vi "Test 1.vi"(8 "error in (no error)":errorcluster, 11 "Test Case In":refnum<class "Tests.lvclass">) -> (0 "error out":errorcluster, 3 "Test Case Out":refnum<class "Tests.lvclass">)   [LabVIEW 2021, in "Tests.lvclass"]
uses:
  Tests.lvclass
  C:/Program Files (x86)/National Instruments/LabVIEW 2021/vi.lib/Astemes/LUnit/Test Case.lvclass
  <vilib>/Astemes/LUnit/Test Case.lvclass/Test Case.ctl
  <vilib>/Astemes/LUnit/Append Fail Result.vi
  <vilib>/Astemes/LUnit/Append Pass Result.vi
  Proto/Hailstone.lvclass
  <vilib>/Astemes/LUnit/Test Case.lvclass
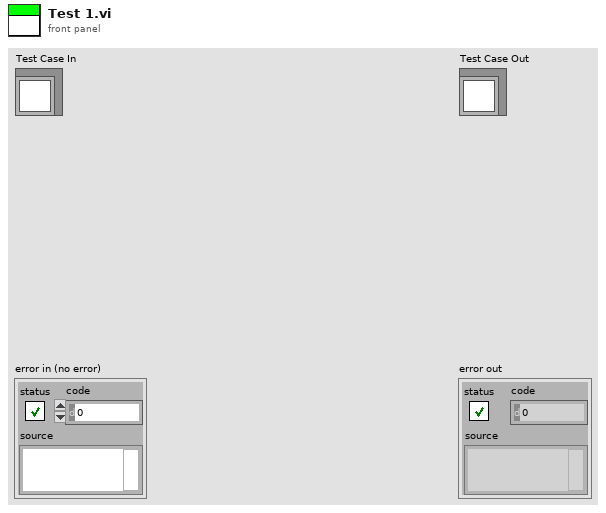
[diagram p1: front panel]
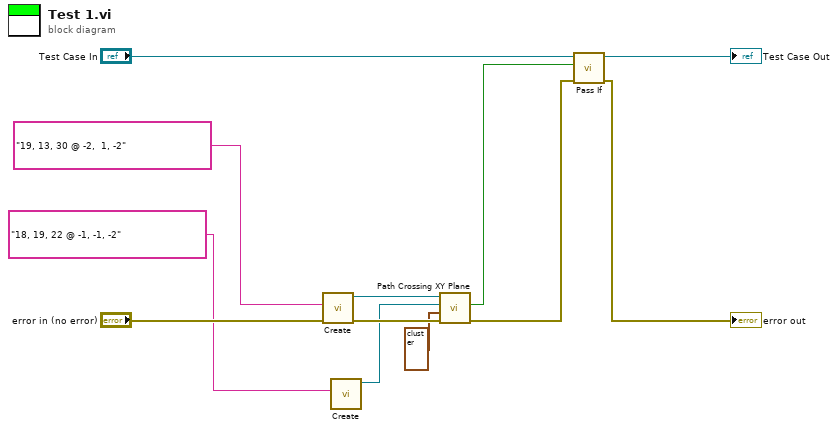
[diagram p0: block diagram]
diagram:
  n1 = call "Create.vi"("error in (no error)"="error in (no error)", "Input"="19, 13, 30 @ -2,  1, -2") -> ("error out"=w8:errorcluster, "Hailstone Out"=w6:refnum<class "Hailstone.lvclass">)  [unwired: 8 in]
  n2 = call "Create.vi"("Input"="18, 19, 22 @ -1, -1, -2") -> ("Hailstone Out"=w3:refnum<class "Hailstone.lvclass">)  [unwired: 9 in, 1 out]
  n3 = call "Path Crossing XY Plane.vi"("error in (no error)"=w8, "Limits"=cluster{"Min":ext, "Max":ext} {"Min"=7.0, "Max"=27.0}, "Hailstone 2"=w3, "Hailstone In"=w6) -> ("error out"=w7:errorcluster, "Crossing?"=w1:bool)  [unwired: 5 in, 1 out]
  n4 = call <vilib>:"Pass If.vi"("error in (no error)"=w7, "Pass?"=w1, "LUnit Test Case In"="Test Case In") -> ("error out"=→"error out":errorcluster, "LUnit Test Case Out"=→"Test Case Out":refnum<class "Tests.lvclass">)  [unwired: 7 in]
